vi "Detector_COM.vi"(8 "error in (no error)":errorcluster, 10 "Selector":string(combo)) -> (0 "error out":errorcluster, 2 "find list":string[](array[string]))   [LabVIEW 2025]
doc: "Detecta los puertos seriales de la computadora y los despliega en un arreglo de Strings"
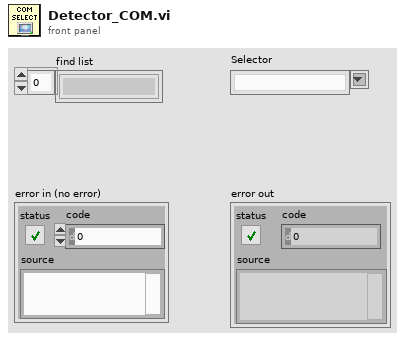
[diagram p1: front panel]
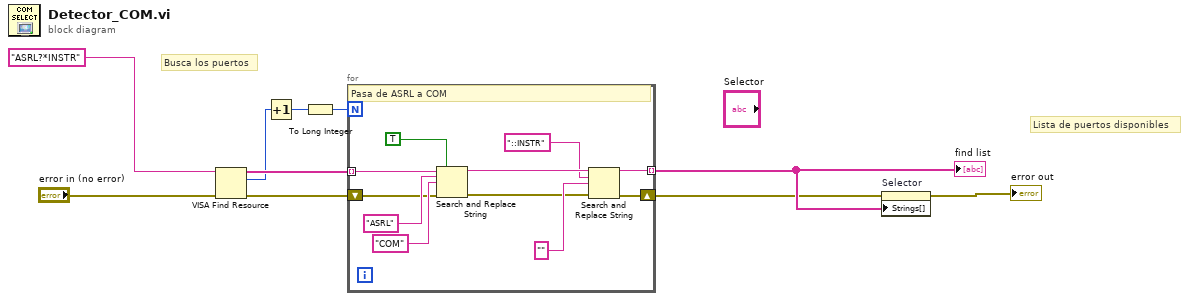
[diagram p0: block diagram]
diagram:
  # "Lista de puertos disponibles"
  # "Busca los puertos"
  n1 = VISA Find Resource(8:"error in (no error)", 11:"ASRL?*INSTR" ("expression (\"?*\")")) -> (0:w8:errorcluster, 2:w5:u32, 3:w9:string[])  [unwired: 1 in]
  n2 = Increment(x=w5) -> (x+1=w4:u32)
  n3 = To Long Integer(number=w4) -> (32bit integer=w3:i32)
  n4 = for {
    N: w3 -> [_]
    tunnel: w9 -> [w18] mode=indexing
    tunnel: [w12] -> w6 mode=indexing
    shift-right: [w11] -> w1
    shift-left: w8 -> [w14]
    # "Pasa de ASRL a COM"
    n5 = Search and Replace String(replace all?=TRUE ("replace all? (F)"), input string=w18, search string="ASRL", replace string="COM" ("replace string (\"\")"), error in=w14) -> (result string=w17:string, error out=w13:errorcluster)  [unwired: 3 in, 2 out]
    n6 = Search and Replace String(input string=w17, search string="::INSTR", replace string="" ("replace string (\"\")"), error in=w13) -> (result string=w12:string, error out=w11:errorcluster)  [unwired: 4 in, 2 out]
  }
  "find list" <- w6
  n7 = property on="Selector" class="CmbBox"(error in=w1, "Strings[]"=w6) -> (error out=→"error out":errorcluster)  [unwired: 1 in, 1 out]
